vi "Initialize Tree with Plugins.vi"(8 "error in (no error)":errorcluster, 11 "Application Data in":T1) -> (0 "error out":errorcluster, 3 "Application Data out":T1)   [LabVIEW 2017, in "DSF Configuration Utility.lvlib"]
uses:
  DSF Configuration Utility.lvlib
  Item Tree/Tree Item.ctl
  View Mode.ctl
  Application Data.ctl
  VeriStand/Data Sharing Custom Device/Source/DSF Core.lvlibp/Classes/Configuration/Configuration Session.lvclass
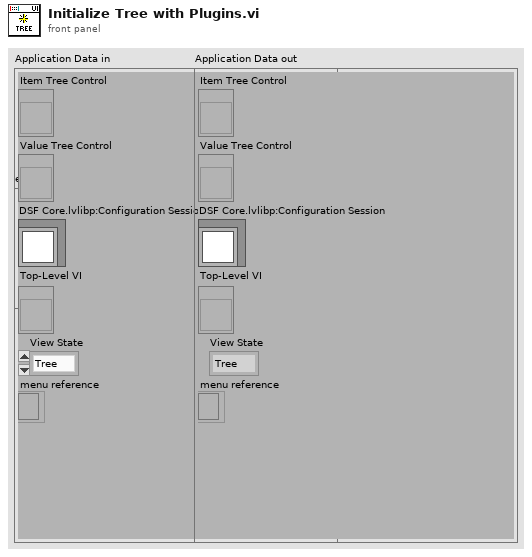
[diagram p1: front panel]
types:
  T1 = typedef "DSF Configuration Utility.lvlib/Application Data.ctl" = cluster{"Item Tree Control":refnum<vi>, "Value Tree Control":refnum<vi>, "DSF Core.lvlibp:Configuration Session":refnum<class "Configuration Session.lvclass">, "Top-Level VI":refnum<vi>, "View State":T2, "menu reference":refnum<k9>}
  T2 = typedef "DSF Configuration Utility.lvlib/View Mode.ctl" = enum16{"Tree", "List"}
  T3 = typedef "DSF Configuration Utility.lvlib/Tree Item.ctl" = cluster{"Left Cell String":string, "Child Text":string[], "Child Tag":string, "Glyph Index":i32}
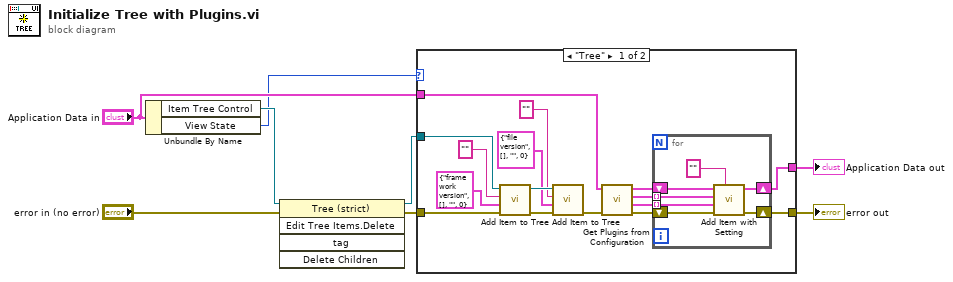
[diagram p0: block diagram]
diagram:
  n1 = Unbundle By Name("Application Data in") -> ("Item Tree Control"=w2:refnum<vi>, "View State"=w1:T2)
  n2 = invoke class="Tree (strict)" method="Edit Tree Items.Delete"(reference=w2, error in="error in (no error)") -> (reference out=w5:refnum<vi>, error out=w6:errorcluster)  [unwired: 3 in, 3 out]
  n3 = case shown="\"Tree\"" w1 {
    tunnel: "Application Data in" -> [w24 w33]
    tunnel: w6 -> [w23 w32]
    tunnel: w5 -> [w14 _]
    tunnel: [w19 w32] -> w4
    tunnel: [w21 w33] -> w3
    frame "Tree" {
      n4 = call "Add Item to Tree.vi"("error in (no error)"=w23, "Item"=T3 {"Left Cell String"="framework version", "Child Text"=[], "Child Tag"="", "Glyph Index"=0}, "parent tag"="", "TreeControl in"=w14) -> ("error out"=w15:errorcluster, "TreeControl out"=w13:refnum<vi>)  [unwired: 5 in, 1 out]
      n5 = call "Add Item to Tree.vi"("error in (no error)"=w15, "Item"=T3 {"Left Cell String"="file version", "Child Text"=[], "Child Tag"="", "Glyph Index"=0}, "parent tag"="", "TreeControl in"=w13) -> ("error out"=w16:errorcluster)  [unwired: 5 in, 2 out]
      n6 = call "Get Plugins from Configuration.vi"("error in (no error)"=w16, "Application Data In"=w24) -> ("error out"=w20:errorcluster, "Settings Items"=w17:T3[], "Plugin Items"=w18:T3[], "Application Data out"=w22:T1)  [unwired: 6 in]
      n7 = for {
        shift-right: [w30] -> w21
        shift-left: w22 -> [w31]
        shift-right: [w28] -> w19
        shift-left: w20 -> [w29]
        tunnel: w18 -> [w26] mode=indexing
        tunnel: w17 -> [w25] mode=indexing
        n8 = call "Add Item with Setting.vi"("Tag"="", "error in (no error)"=w29, "Setting"=w25, "Item"=w26, "Application Data in"=w31) -> ("error out"=w28:errorcluster, "Application Data out"=w30:T1)  [unwired: 4 in, 1 out]
      }
    }
    frame "List" {
    }
  }
  "error out" <- w4
  "Application Data out" <- w3
